vi "Get Children Items.vi"(8 "error in (no error)":errorcluster, 10 "Whole Hierarchy?(F)":bool, 11 "Section Reference in":u64 format="%.0x") -> (0 "error out":errorcluster, 1 "Children Item Names":string[](array[string]), 2 "Children Item References":u64[](array[numeric]) format="%.0x", 3 "Section Reference out":u64 format="%.0x", 4 "found":bool)   [LabVIEW 2013, in "Hierarchy Framework.lvlib" / "Section.lvclass"]
doc: "It will get all the children items if the <b>Whole Hierarchy</b> is <b>True</b>."
uses:
  Section.lvclass
  Generic/Generic.lvclass
  Item/Item.lvclass
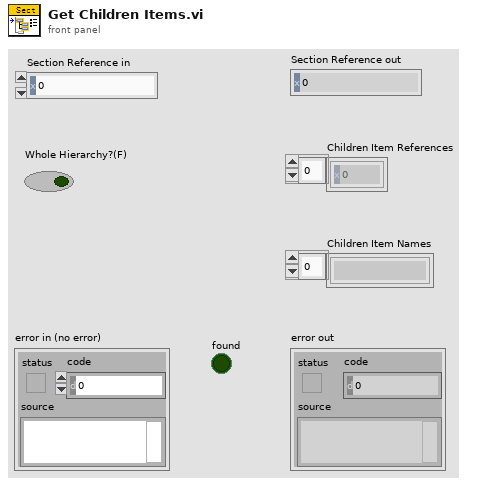
[diagram p1: front panel]
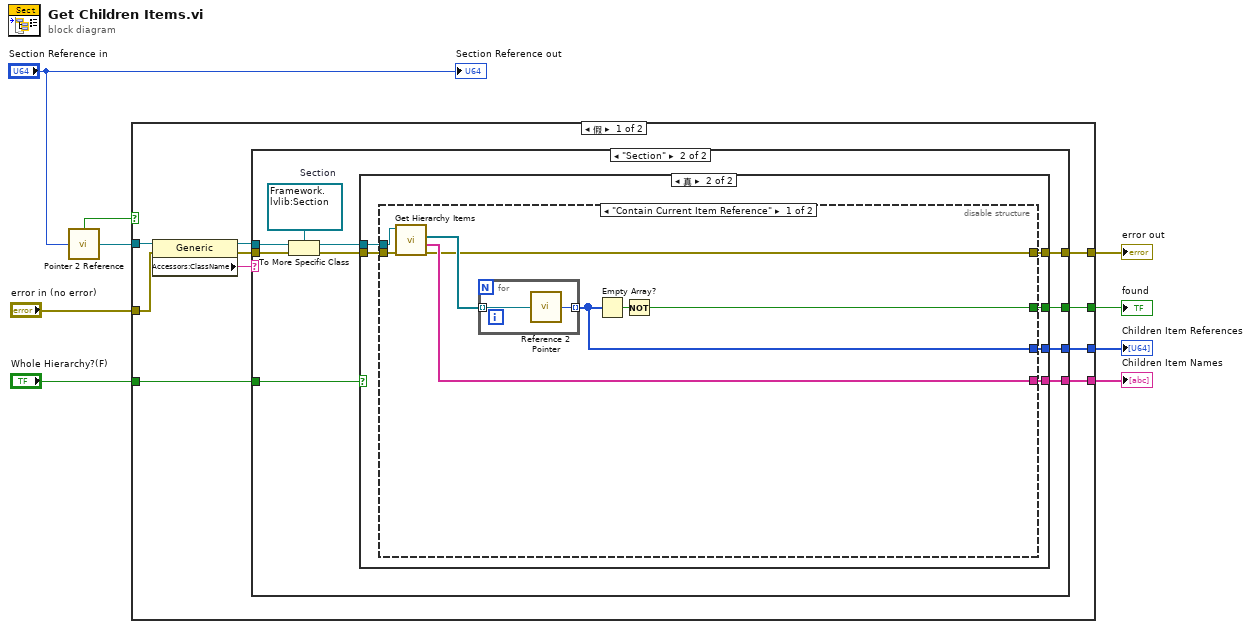
[diagram p0: block diagram]
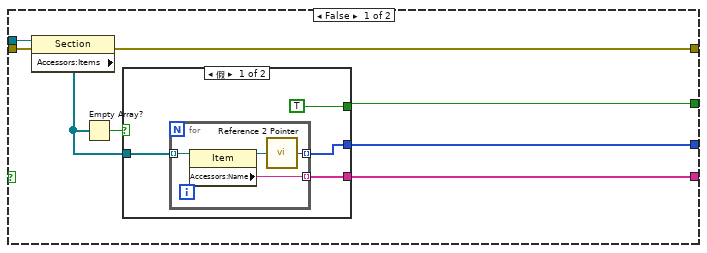
[diagram p3: hidden frame]
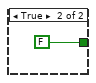
[diagram p4: hidden frame]
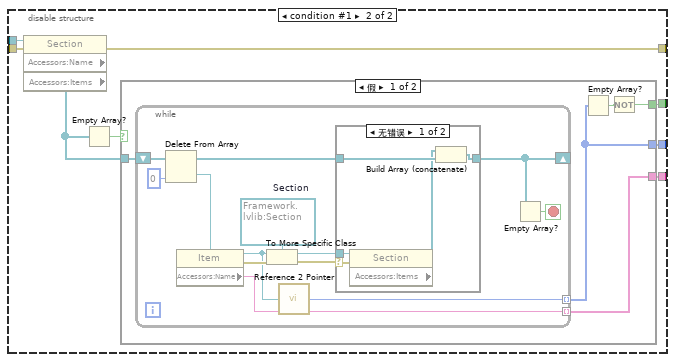
[diagram p5: hidden frame]
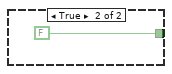
[diagram p7: hidden frame]
diagram:
  n1 = call "Pointer 2 Reference.vi"("Pointer"="Section Reference in") -> ("Not A Refnum?"=w6:bool, "Generic Reference"=w5:refnum<data-value>)
  n2 = case shown="假" w6 {
    tunnel: w5 -> [w18 _]
    tunnel: "error in (no error)" -> [w17 w97]
    tunnel: [w19 w97] -> w8
    tunnel: [w13 _] -> w3
    tunnel: [w12 _] -> w4
    tunnel: [w11 _] -> w2
    tunnel: "Whole Hierarchy?(F)" -> [w10 _]
    frame False {
      n3 = property class="Generic"(reference=w18, error in=w17) -> (reference out=w15:refnum<data-value>, error out=w16:errorcluster, "Accessors:ClassName"=w14:string)
      n4 = case shown="\"Section\"" w14 {
        tunnel: [w20 w25] -> w19
        tunnel: w16 -> [w20 w27]
        tunnel: w15 -> [_ w26]
        tunnel: [_ w24] -> w13
        tunnel: [_ w23] -> w12
        tunnel: [_ w22] -> w11
        tunnel: w10 -> [_ w21]
        frame Default {
        }
        frame "Section" {
          w30 = refnum<data-value> refnum  # Section
          n5 = To More Specific Class(target class=w30, reference=w26, error in=w27) -> (specific class reference=w29:refnum<data-value>, error out=w28:errorcluster)
          n6 = case shown="真" w21 {
            tunnel: w29 -> [w38 w53]
            tunnel: w28 -> [w37 w52]
            tunnel: [w36 w50] -> w25
            tunnel: [w33 w49] -> w24
            tunnel: [w32 w48] -> w23
            tunnel: [w31 w51] -> w22
            frame False {
              n7 = property class="Section"(reference=w38, error in=w37) -> (error out=w36:errorcluster, "Accessors:Items"=w35:refnum<data-value>[])  [unwired: 1 out]
              n8 = Empty Array?(array=w35) -> (empty?=w34:bool)
              n9 = case shown="假" w34 {
                tunnel: w35 -> [w42 _]
                tunnel: [w41 _] -> w33
                tunnel: [TRUE FALSE] -> w32
                tunnel: [w39 _] -> w31
                frame False {
                  n10 = for {
                    tunnel: w42 -> [w46] mode=indexing
                    tunnel: [w45] -> w39 mode=indexing
                    tunnel: [w43] -> w41 mode=indexing
                    n11 = property class="Item"(reference=w46) -> (reference out=w44:refnum<data-value>, "Accessors:Name"=w45:string)  [unwired: 1 in, 1 out]
                    n12 = call "Reference 2 Pointer.vi"("Generic Reference"=w44) -> ("Pointer"=w43:u64)  [unwired: 1 out]
                  }
                }
                frame True {
                }
              }
            }
            frame True {
              n13 = disable-structure shown="\"Contain Current Item Reference\"" {
                disable-tunnel: w53 -> [w61 w71]
                disable-tunnel: w52 -> [w60 w70]
                disable-tunnel: [w59 w64] -> w51
                disable-tunnel: [w57 w66] -> w50
                disable-tunnel: [w56 w67] -> w49
                disable-tunnel: [w54 w65] -> w48
                frame condition #0 (active) {
                  n14 = call "Get Hierarchy Items.vi"("错误输入（无错误）"=w60, "Section in"=w61) -> ("错误输出"=w57:errorcluster, "Names"=w59:string[], "Items"=w58:refnum<data-value>[])  [unwired: 6 in, 1 out]
                  n15 = for {
                    tunnel: w58 -> [w63] mode=indexing
                    tunnel: [w62] -> w56 mode=indexing
                    n16 = call "Reference 2 Pointer.vi"("Generic Reference"=w63) -> ("Pointer"=w62:u64)  [unwired: 1 out]
                  }
                  n17 = Empty Array?(array=w56) -> (empty?=w55:bool)
                  n18 = Not(x=w55) -> (.not. x?=w54:bool)
                }
                frame condition #1 {
                  n19 = property class="Section" props=["Accessors:Name", "Accessors:Items"](reference=w71, error in=w70) -> (error out=w66:errorcluster, "Accessors:Items"=w68:refnum<data-value>[])  [unwired: 2 out]
                  n20 = Empty Array?(array=w68) -> (empty?=w69:bool)
                  n21 = case shown="假" w69 {
                    tunnel: w68 -> [w76 _]
                    tunnel: [w72 _] -> w67
                    tunnel: [w73 FALSE] -> w65
                    tunnel: [w75 _] -> w64
                    frame False {
                      n22 = while {
                        shift-right: [w77] -> _
                        shift-left: w76 -> [w89]
                        tunnel: [w80] -> w75 mode=indexing
                        tunnel: [w78] -> w72 mode=indexing
                        stop <- w82 stop-if-true
                        w85 = refnum<data-value> refnum  # Section
                        n23 = Delete From Array(array=w89, index=0 ("索引")) -> (deleted portion=w87:refnum<data-value>, array with subset deleted=w81:refnum<data-value>[])  [unwired: 1 in]
                        n24 = property class="Item"(reference=w87) -> (reference out=w79:refnum<data-value>, error out=w86:errorcluster, "Accessors:Name"=w80:string)  [unwired: 1 in]
                        n25 = To More Specific Class(target class=w85, reference=w79, error in=w86) -> (specific class reference=w83:refnum<data-value>, error out=w84:errorcluster)
                        n26 = call "Reference 2 Pointer.vi"("Generic Reference"=w79) -> ("Pointer"=w78:u64)  [unwired: 1 out]
                        n27 = case shown="无错误" w84 {
                          selector: w84 -> [w93 _]
                          tunnel: w83 -> [w94 _]
                          tunnel: w81 -> [w92 w95]
                          tunnel: [w90 w95] -> w77
                          frame No Error {
                            n28 = property class="Section"(reference=w94, error in=w93) -> ("Accessors:Items"=w91:refnum<data-value>[])  [unwired: 2 out]
                            n29 = Build Array (concatenate)(w91, w92) -> (w90:refnum<data-value>[])
                          }
                          frame Error {
                          }
                        }
                        n30 = Empty Array?(array=w77) -> (empty?=w82:bool)
                      }
                      n31 = Empty Array?(array=w72) -> (empty?=w74:bool)
                      n32 = Not(x=w74) -> (.not. x?=w73:bool)
                    }
                    frame True {
                    }
                  }
                }
              }
            }
          }
        }
      }
    }
    frame True {
    }
  }
  "error out" <- w8
  "found" <- w4
  "Children Item References" <- w3
  "Children Item Names" <- w2
  "Section Reference out" <- "Section Reference in"
